vi "parabola fitZ.vi"(8 "radial profile":dbl[](array[numeric])) -> (0 "Y focus":dbl)   [LabVIEW 2011, in "OfflineTracker.lvlib"]
uses:
  OfflineTracker.lvlib
  <vilib>/Analysis/NI_AALPro.lvlib
panel:
  out "Waveform Graph 2":dbl[](graph)
  out "Waveform Graph":dbl[](graph)
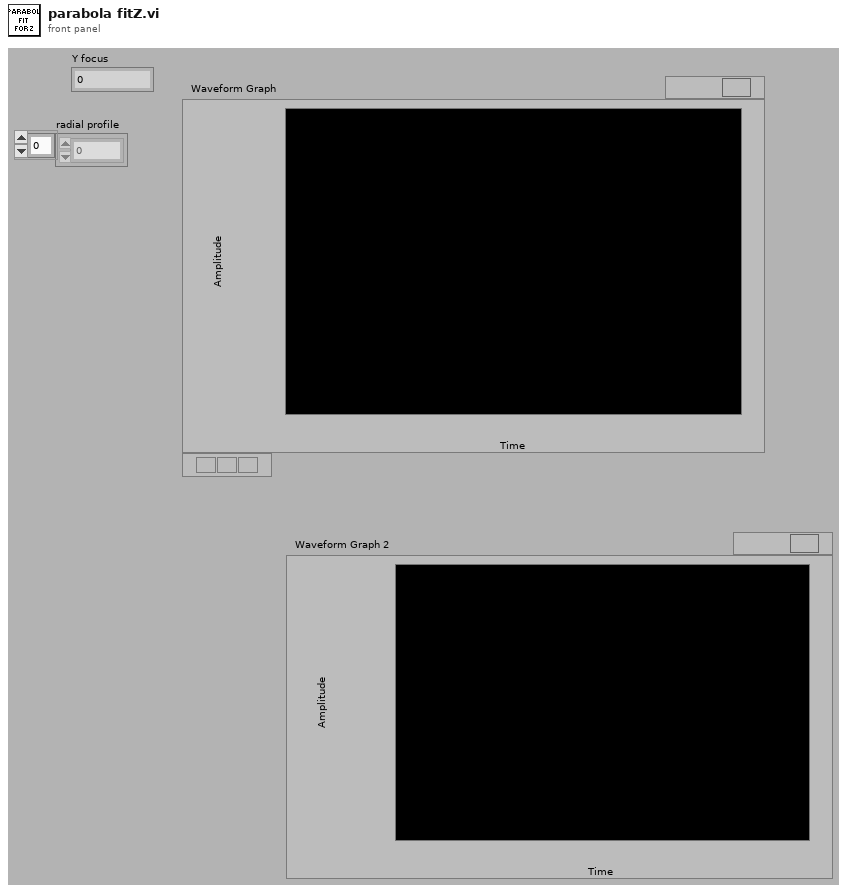
[diagram p1: front panel]
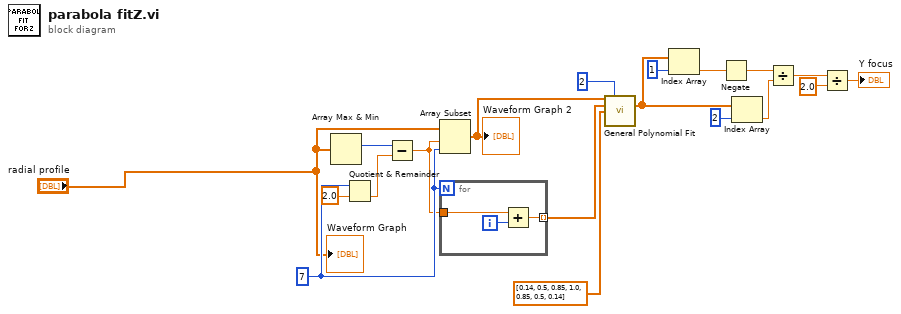
[diagram p0: block diagram]
diagram:
  w8 = 7 ("index")
  n1 = Array Max & Min(array="radial profile") -> (max index (indices)=w16:i32)  [unwired: 3 out]
  n2 = Quotient & Remainder(x=w8, y=2.0) -> (floor(x/y)=w9:dbl)  [unwired: 1 out]
  n3 = Subtract(x=w16, y=w9) -> (x-y=w6:dbl)
  n4 = Array Subset(array="radial profile", index=w6, length=w8) -> (w2:dbl[])
  "Waveform Graph 2" <- w2
  n5 = for {
    N: w8 -> [_]
    tunnel: [w21] -> w3 mode=indexing
    tunnel: w6 -> [w20]
    i -> [w22]
    n6 = Add(x=w20, y=w22) -> (x+y=w21:dbl)
  }
  n7 = call <vilib>:"General Polynomial Fit.vi"("Y"=w2, "polynomial order"=2, "X"=w3, "Weight"=dbl[] [0.14, 0.5, 0.85, 1.0, 0.85, 0.5, 0.14] ("X")) -> ("Polynomial Coefficients"=w4:dbl[])  [unwired: 8 in, 3 out]
  n8 = Index Array(array=w4, index=1 ("Index")) -> (element=w12:dbl)
  n9 = Negate(x=w12) -> (-x=w10:dbl)
  n10 = Index Array(array=w4, index=2 ("Index")) -> (element=w11:dbl)
  n11 = Divide(x=w10, y=w11) -> (x/y=w14:dbl)
  n12 = Divide(x=w14, y=2.0) -> (x/y=→"Y focus":dbl)
  "Waveform Graph" <- "radial profile"
